vi "Write Data.vi"(8 "error in":errorcluster, 10 "Quaternion":T1) -> (0 "error out":errorcluster, 3 "Orient3d out":refnum<class "Orient3d Class.lvclass">)   [LabVIEW 2017, in "Orient3d Class.lvclass"]
uses:
  Orient3d Class.lvclass
  Type Definitions/Quaternion.ctl
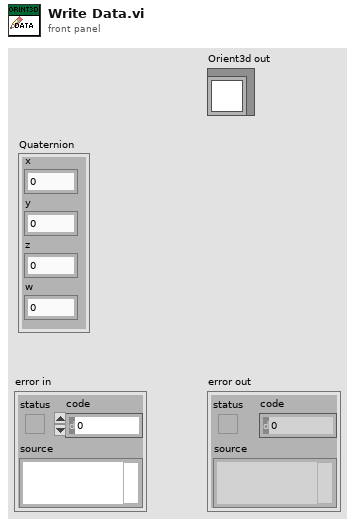
[diagram p1: front panel]
types:
  T1 = typedef "Quaternion.ctl" = cluster{"x":dbl, "y":dbl, "z":dbl, "w":dbl}
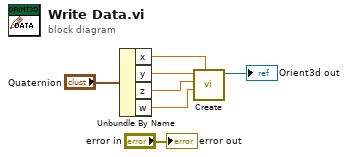
[diagram p0: block diagram]
diagram:
  n1 = Unbundle By Name("Quaternion") -> ("x"=w5:dbl, "y"=w4:dbl, "z"=w3:dbl, "w"=w2:dbl)
  n2 = call "Create.vi"("x"=w5, "w"=w2, "z"=w3, "y"=w4) -> ("Orient3d out"=→"Orient3d out":refnum<class "Orient3d Class.lvclass">)  [unwired: 6 in, 1 out]
  "error out" <- "error in"
